vi "Cancel.vi"(8 "error in (no error)":errorcluster, 9 "Cancel":bool=TRUE) -> (0 "error out":errorcluster)   [LabVIEW 2014, in "Utilities.lvlib"]
uses:
  Utilities.lvlib
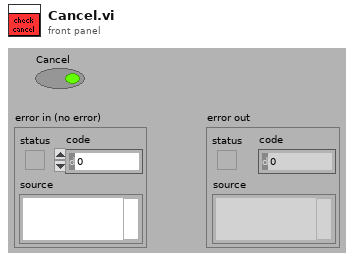
[diagram p1: front panel]
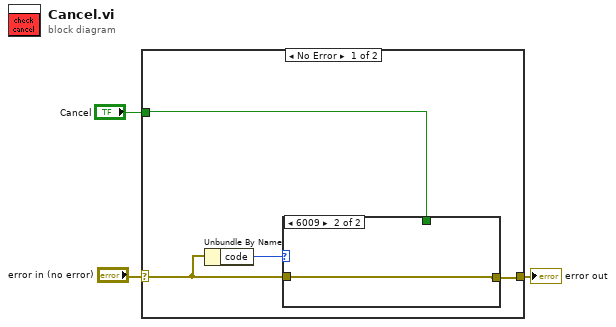
[diagram p0: block diagram]
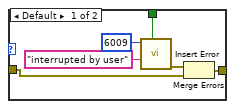
[diagram p2: hidden frame]
diagram:
  n1 = case shown="No Error" "error in (no error)" {
    selector: "error in (no error)" -> [w5 w15]
    tunnel: [w6 w15] -> w2
    tunnel: "Cancel" -> [w7 _]
    frame No Error {
      n2 = Unbundle By Name(w5) -> ("code"=w4:i32)
      n3 = case shown="6009" w4 {
        tunnel: w7 -> [w13 _]
        tunnel: [w9 w14] -> w6
        tunnel: w5 -> [w8 w14]
        frame Default {
          n4 = call "Insert Error.vi"("[error code] (0)"=6009, "error description"="interrupted by user", "error?"=w13) -> ("error out"=w10:errorcluster)  [unwired: 7 in]
          n5 = Merge Errors(w10, w8) -> (w9:errorcluster)
        }
        frame 6009 {
        }
      }
    }
    frame Error {
    }
  }
  "error out" <- w2
